vi "SwerveDriveOpenSensors.vi"(0 "SwerveDriveDevRef":T2={"DevStatus"={"status"=FALSE, "code"=0, "source"=""}, "TurnMotors[]"=[], "Square Inputs"=FALSE, "Max Output"=1.0, "DriveMotors[]"=[], "WheelOffset[]"=[], "SwerveSensors[]"=[], "RobotSize"={"Width"=[], "Length"=[], "Center"=[]}}, 1 "Rear Left Encoder":T1, 2 "Rear Right Encoder":T1=enum."AI 1", 3 "Front Left Encoder":T1=enum."AI 2", 4 "Front Right Encoder":T1=enum."AI 3", 5 "error in (no error)":errorcluster) -> (14 "SwerveDriveDevRef":T2={"DevStatus"={"status"=FALSE, "code"=0, "source"=""}, "TurnMotors[]"=[], "Square Inputs"=FALSE, "Max Output"=1.0, "DriveMotors[]"=[], "WheelOffset[]"=[], "SwerveSensors[]"=[], "RobotSize"={"Width"=[], "Length"=[], "Center"=[]}}, 19 "error out":errorcluster)   [LabVIEW 2019, in "Swerve Drive.lvlib"]
uses:
  Swerve Drive.lvlib
  SwerveDriveDevRef.ctl
  <vilib>/Rock Robotics/WPI/MotorControl/WPI_MotorControlDeviceRef.ctl
  <vilib>/Rock Robotics/WPI/MotorControl/WPI_MotorControlType.ctl
  <vilib>/Rock Robotics/SystemInterfaces/DIO/FPGA_DIOPWMChannel.ctl
  <vilib>/Rock Robotics/WPI/PWM/WPI_PWMDeadband.ctl
  <vilib>/Rock Robotics/SystemInterfaces/DIO/FPGA_DIOChannel.ctl
  <vilib>/Rock Robotics/SystemInterfaces/AI/FPGA_AIChannel.ctl
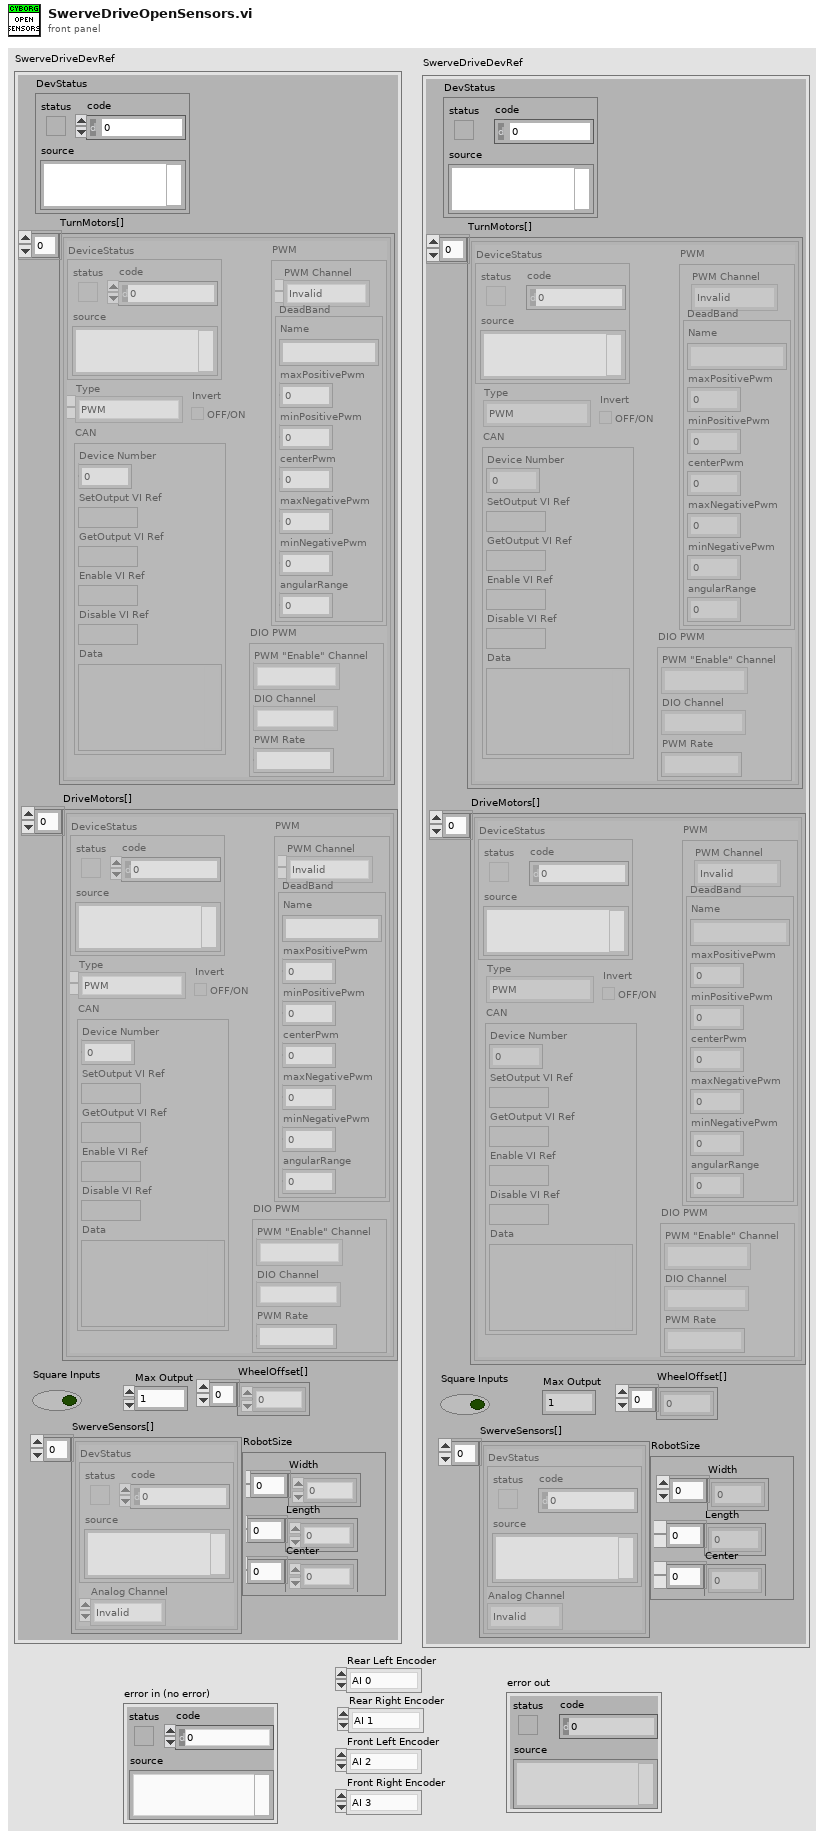
[diagram p1: front panel]
types:
  T1 = typedef "FPGA_AIChannel.ctl" = enum8{"AI 0", "AI 1", "AI 2", "AI 3", "AI MXP 0", "AI MXP 1", "AI MXP 2", "AI MXP 3", "Invalid"}
  T2 = typedef "Swerve Drive.lvlib/SwerveDriveDevRef.ctl" = cluster{"DevStatus":errorcluster, "TurnMotors[]":T3[], "Square Inputs":bool, "Max Output":dbl, "DriveMotors[]":T3[], "WheelOffset[]":dbl[], "SwerveSensors[]":cluster{"DevStatus":errorcluster, "Analog Channel":T1}[], "RobotSize":cluster{"Width":dbl[], "Length":dbl[], "Center":dbl[]}}
  T3 = typedef "WPI_MotorControlDeviceRef.ctl" = cluster{"DeviceStatus":errorcluster, "Type":T4, "PWM":cluster{"PWM Channel":T5, "DeadBand":T6}, "CAN":cluster{"Device Number":u8, "SetOutput VI Ref":variant, "GetOutput VI Ref":variant, "Enable VI Ref":variant, "Disable VI Ref":variant, "Data":variant}, "Invert":bool, "DIO PWM":cluster{"PWM \"Enable\" Channel":T5, "DIOChannel":T7, "PWM Rate":dbl}}
  T4 = typedef "WPI_MotorControlType.ctl" = enum16{"PWM", "CAN", "DIO PWM"}
  T5 = typedef "FPGA_DIOPWMChannel.ctl" = enum8{"PWM 0", "PWM 1", "PWM 2", "PWM 3", "PWM 4", "PWM 5", "PWM 6", "PWM 7", "PWM 8", "PWM 9", "PWM MXP 0", "PWM MXP 1", "PWM MXP 2", "PWM MXP 3", "PWM MXP 4", "PWM MXP 5", "PWM MXP 6", "PWM MXP 7", "PWM MXP 8", "PWM MXP 9", "Invalid"}
  T6 = typedef "WPI_PWMDeadband.ctl" = cluster{"Name":string, "maxPositivePwm":i32, "minPositivePwm":i32, "centerPwm":i32, "maxNegativePwm":i32, "minNegativePwm":i32, "angularRange":u16}
  T7 = typedef "FPGA_DIOChannel.ctl" = enum8{"DIO 0", "DIO 1", "DIO 2", "DIO 3", "DIO 4", "DIO 5", "DIO 6", "DIO 7", "DIO 8", "DIO 9", "DIO MXP 0", "DIO MXP 1", "DIO MXP 2", "DIO MXP 3", "DIO MXP 4", "DIO MXP 5", "DIO MXP 6", "DIO MXP 7", "DIO MXP 8", "DIO MXP 9", "DIO MXP 10", "DIO MXP 11", "DIO MXP 12", "DIO MXP 13", "DIO MXP 14", "DIO MXP 15", "SPI Port CS1", "SPI Port CS2", "SPI Port CS3", "SPI Port MISO", "SPI Port MOSI", "Invalid"}
  T8 = typedef "WPI_AnalogChannelDevRef.ctl" = cluster{"DevStatus":errorcluster, "Analog Channel":T1}
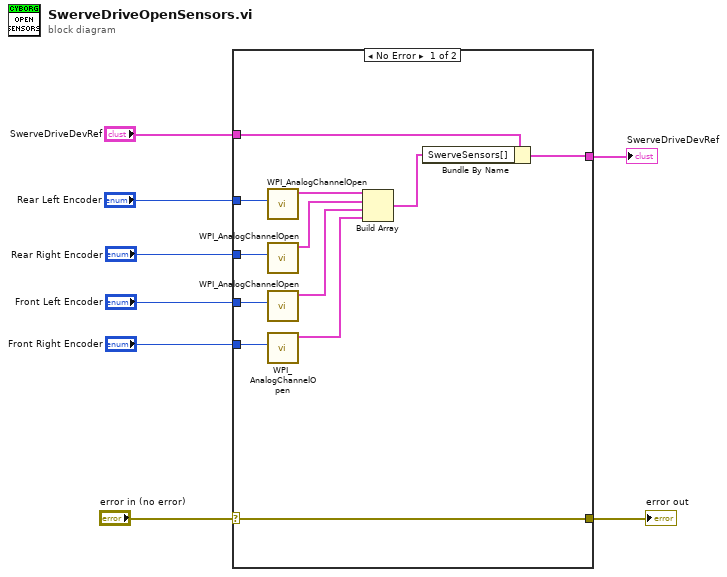
[diagram p0: block diagram]
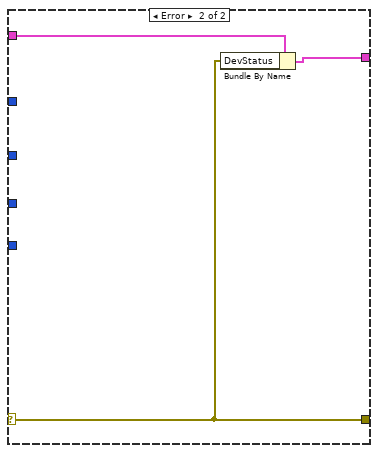
[diagram p2: hidden frame]
diagram:
  n1 = case shown="No Error" "error in (no error)" {
    selector: "error in (no error)" -> [w20 w21]
    tunnel: [w20 w21] -> w7
    tunnel: "SwerveDriveDevRef" -> [w18 w23]
    tunnel: [w19 w22] -> w5
    tunnel: "Rear Left Encoder" -> [w12 _]
    tunnel: "Front Right Encoder" -> [w11 _]
    tunnel: "Front Left Encoder" -> [w10 _]
    tunnel: "Rear Right Encoder" -> [w9 _]
    frame No Error {
      n2 = call <vilib>:"WPI_AnalogChannelOpen.vi"("Analog Channel"=w12) -> ("AIDeviceRef"=w16:T8)  [unwired: 9 in, 1 out]
      n3 = call <vilib>:"WPI_AnalogChannelOpen.vi"("Analog Channel"=w9) -> ("AIDeviceRef"=w15:T8)  [unwired: 9 in, 1 out]
      n4 = call <vilib>:"WPI_AnalogChannelOpen.vi"("Analog Channel"=w10) -> ("AIDeviceRef"=w14:T8)  [unwired: 9 in, 1 out]
      n5 = call <vilib>:"WPI_AnalogChannelOpen.vi"("Analog Channel"=w11) -> ("AIDeviceRef"=w13:T8)  [unwired: 9 in, 1 out]
      n6 = Build Array(w16, w15, w14, w13) -> (w17:T8[])
      n7 = Bundle By Name(cluster=w18, "SwerveSensors[]"=w17) -> (w19:T2)
    }
    frame Error {
      n8 = Bundle By Name(cluster=w23, "DevStatus"=w21) -> (w22:T2)
    }
  }
  "SwerveDriveDevRef" <- w5
  "error out" <- w7
